vi "_Build_Cluster_Query.vi"(8 "error in (no error)":errorcluster, 11 "Postgres Connector In":refnum<class "Postgres Connector.lvclass">) -> (0 "error out":errorcluster, 1 "State After Query":string, 2 "Query Return":T1, 3 "Postgres Connector Out":refnum<class "Postgres Connector.lvclass">)   [LabVIEW 2020, in "Postgres Connector.lvclass"]
doc: "This VI build the cluster containing the important information of the query"
uses:
  Postgres Connector.lvclass
  Cluster_Return_Of_The_Query.ctl
  Postgres Connector.lvclass/Postgres Connector.ctl
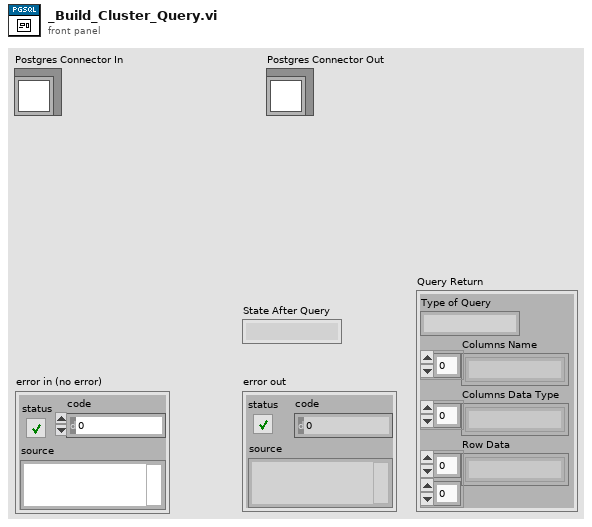
[diagram p1: front panel]
types:
  T1 = typedef "Postgres Connector.lvclass/Cluster_Return_Of_The_Query.ctl" = cluster{"Type of Query":string, "Columns Name":string[], "Columns Data Type":string[], "Row Data":string[][]}
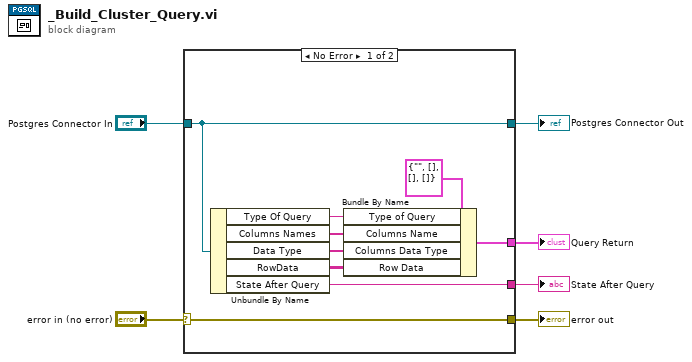
[diagram p0: block diagram]
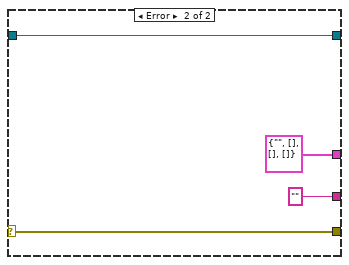
[diagram p2: hidden frame]
diagram:
  n1 = case shown="No Error" "error in (no error)" {
    selector: "error in (no error)" -> [w13 w19]
    tunnel: [w14 T1 {"Type of Query"="", "Columns Name"=[], "Columns Data Type"=[], "Row Data"=[]}] -> w6
    tunnel: [w13 w19] -> w4
    tunnel: "Postgres Connector In" -> [w7 w16]
    tunnel: [w9 "" ("State After Query")] -> w2
    tunnel: [w7 w16] -> w1
    frame No Error {
      n2 = Unbundle By Name(w7) -> ("Type Of Query"=w8:string, "Columns Names"=w10:string[], "Data Type"=w12:string[], "RowData"=w11:string[][], "State After Query"=w9:string)
      n3 = Bundle By Name(cluster=T1 {"Type of Query"="", "Columns Name"=[], "Columns Data Type"=[], "Row Data"=[]}, "Type of Query"=w8, "Columns Name"=w10, "Columns Data Type"=w12, "Row Data"=w11) -> (w14:T1)
    }
    frame Error {
    }
  }
  "error out" <- w4
  "Query Return" <- w6
  "State After Query" <- w2
  "Postgres Connector Out" <- w1
